vi "Power Off Dut.vi"(8 "error in":errorcluster, 11 "Power Sequencing File Path":path) -> (0 "error out":errorcluster)   [LabVIEW 2023]
uses:
  NI gRPC Device Server - Action.ctl
  <instrlib>/niDCPower/nidcpower.llb/niDCPower gRPC Device Server.ctl
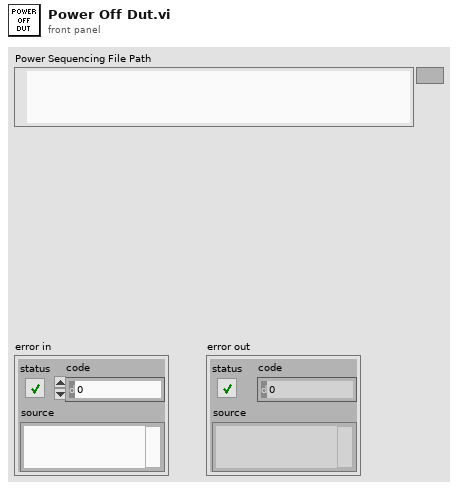
[diagram p1: front panel]
types:
  T1 = typedef "NI gRPC Device Server - Action.ctl" = enum16{"Start Server", "End Server"}
  T2 = typedef "DC Ins Initialize.ctl" = cluster{"Pin Name":string, "Resource Name":refnum<k15>, "Channel":string, "Voltage Range (V)":dbl, "Current Range (A)":dbl}
  T3 = typedef "DC Settings.ctl" = cluster{"Pin Name":string, "Resource Name":refnum<k15>, "Channel":string, "Power-up Seq":u32, "Power-up Voltage (V)":dbl, "Power-down Seq":u32, "Power-down Voltage (V)":dbl, "Current Limit (A)":dbl, "Wait Before Next (ms)":u32}
  T4 = typedef "niDCPower gRPC Device Server.ctl" = cluster{"session name":string, "address (localhost)":string, "port (31763)":u32}
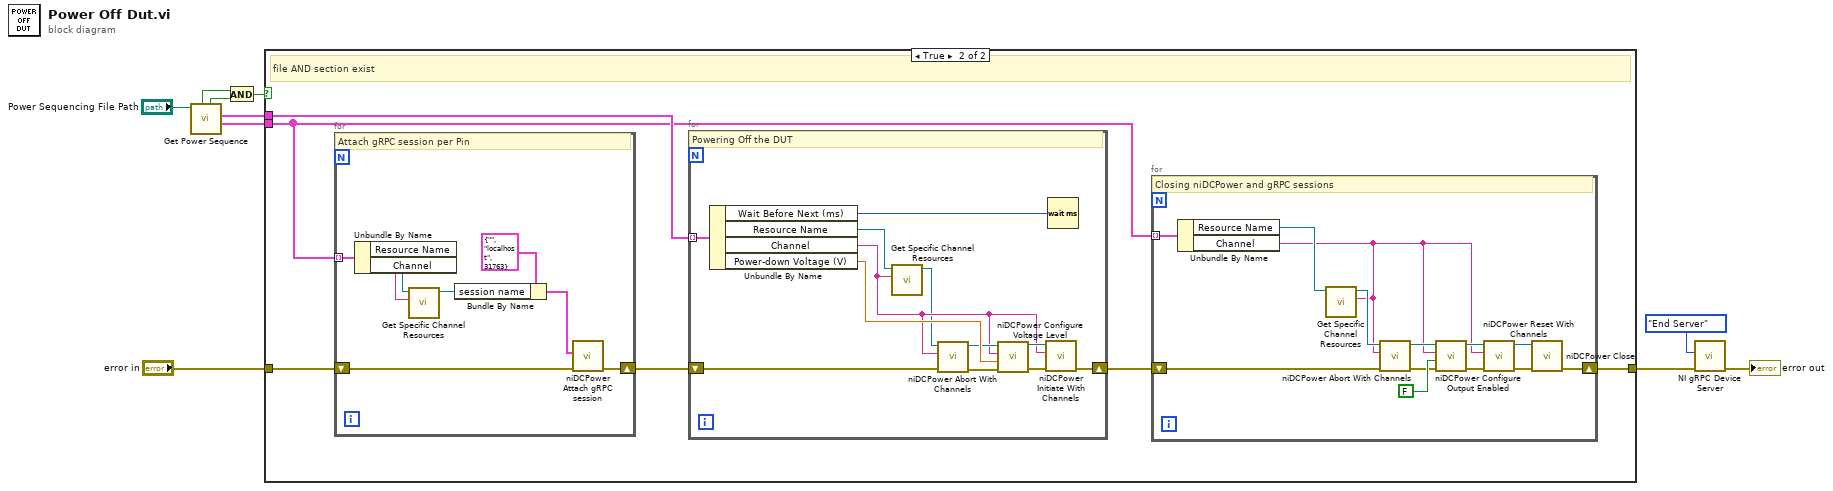
[diagram p0: block diagram]
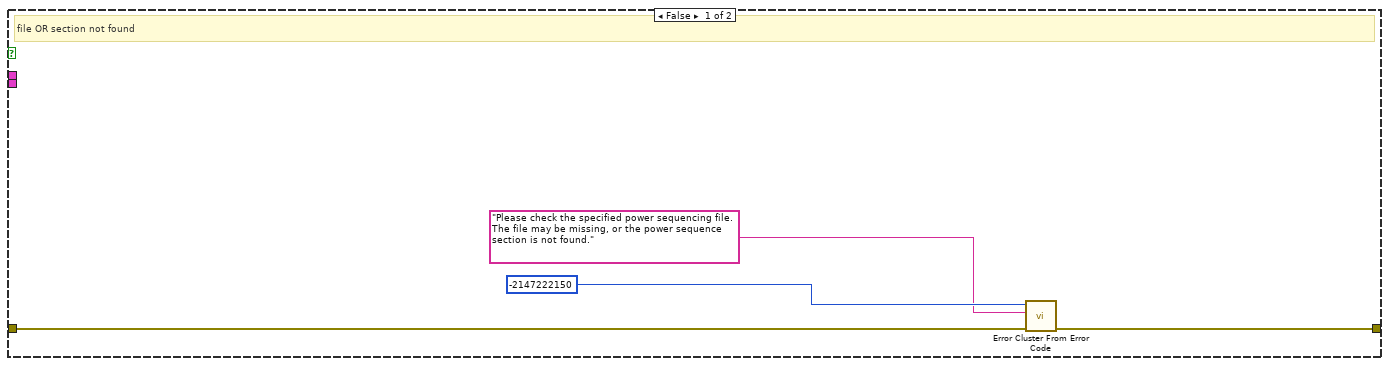
[diagram p2: hidden frame]
diagram:
  n1 = call "Get Power Sequence.vi"("File Path"="Power Sequencing File Path") -> ("SMUs to Initialize (not in order)"=w10:T2[], "Power down Seq"=w9:T3[], "File Exists?"=w6:bool, "Section Exists?"=w5:bool)  [unwired: 6 in, 1 out]
  n2 = And(x=w5, y=w6) -> (x .and. y?=w7:bool)
  n3 = case shown="True" w7 {
    tunnel: w10 -> [_ w16]
    tunnel: w9 -> [_ w20]
    tunnel: "error in" -> [w12 w17]
    tunnel: [w11 w18] -> w3
    frame False {
      # "file OR section not found"
      n4 = call <vilib>:"Error Cluster From Error Code.vi"("error in (no error)"=w12, "error message (\"\")"="Please check the specified power sequencing file. The file may be missing, or the power sequence section is not found.", "error code (0)"=-2147222150) -> ("error out"=w11:errorcluster)  [unwired: 6 in]
    }
    frame True {
      # "file AND section exist"
      n5 = for {
        tunnel: w16 -> [w28] mode=indexing
        shift-right: [w21] -> w15
        shift-left: w17 -> [w22]
        # "Attach gRPC session per Pin"
        n6 = Unbundle By Name(w28) -> ("Resource Name"=w27:refnum<k15>, "Channel"=w26:string)
        n7 = call "Get Specific Channel Resources.vi"("Channel"=w26, "Resource Name"=w27) -> ("Resource Name"=w24:refnum<k15>)  [unwired: 9 in]
        n8 = Bundle By Name(cluster=T4 {"session name"="", "address (localhost)"="localhost", "port (31763)"=31763} ("gRPC options"), "session name"=w24) -> (w23:T4)
        n9 = call <instrlib>:"niDCPower Attach gRPC session.vi"("error in (no error)"=w22, "gRPC options"=w23) -> ("error out"=w21:errorcluster)  [unwired: 8 in, 1 out]
      }
      n10 = for {
        tunnel: w20 -> [w38] mode=indexing
        shift-right: [w33] -> w19
        shift-left: w15 -> [w30]
        # "Powering Off the DUT"
        n11 = Unbundle By Name(w38) -> ("Wait Before Next (ms)"=w39:u32, "Resource Name"=w40:refnum<k15>, "Channel"=w31:string, "Power-down Voltage (V)"=w37:dbl)
        n12 = call "Get Specific Channel Resources.vi"("Channel"=w31, "Resource Name"=w40) -> ("Resource Name"=w29:refnum<k15>)  [unwired: 9 in]
        n13 = call <instrlib>:"niDCPower Abort With Channels.vi"("error in (no error)"=w30, "channel name"=w31, "instrument handle"=w29) -> ("error out"=w36:errorcluster, "instrument handle out"=w35:refnum<k15>)  [unwired: 7 in]
        n14 = call <instrlib>:"niDCPower Configure Voltage Level.vi"("error in (no error)"=w36, "voltage level"=w37, "channel name"=w31, "instrument handle"=w35) -> ("error out"=w34:errorcluster, "instrument handle out"=w32:refnum<k15>)  [unwired: 6 in]
        n15 = call <instrlib>:"niDCPower Initiate With Channels.vi"("error in (no error)"=w34, "channel name"=w31, "instrument handle"=w32) -> ("error out"=w33:errorcluster)  [unwired: 7 in, 1 out]
        n16 = Wait (ms)(milliseconds to wait=w39) -> ()  [unwired: 1 out]
      }
      n17 = for {
        tunnel: w16 -> [w50] mode=indexing
        shift-right: [w41] -> w18
        shift-left: w19 -> [w47]
        # "Closing niDCPower and gRPC sessions"
        n18 = Unbundle By Name(w50) -> ("Resource Name"=w53:refnum<k15>, "Channel"=w42:string)
        n19 = call "Get Specific Channel Resources.vi"("Channel"=w42, "Resource Name"=w53) -> ("Resource Name"=w48:refnum<k15>)  [unwired: 9 in]
        n20 = call <instrlib>:"niDCPower Abort With Channels.vi"("error in (no error)"=w47, "channel name"=w42, "instrument handle"=w48) -> ("error out"=w45:errorcluster, "instrument handle out"=w46:refnum<k15>)  [unwired: 7 in]
        n21 = call <instrlib>:"niDCPower Configure Output Enabled.vi"("error in (no error)"=w45, "output enabled"=FALSE, "channel name"=w42, "instrument handle"=w46) -> ("error out"=w43:errorcluster, "instrument handle out"=w44:refnum<k15>)  [unwired: 6 in]
        n22 = call <instrlib>:"niDCPower Reset With Channels.vi"("error in (no error)"=w43, "channel name"=w42, "instrument handle"=w44) -> ("error out"=w51:errorcluster, "instrument handle out"=w52:refnum<k15>)  [unwired: 7 in]
        n23 = call <instrlib>:"niDCPower Close.vi"("error in (no error)"=w51, "instrument handle"=w52) -> ("error out"=w41:errorcluster)  [unwired: 9 in]
      }
    }
  }
  n24 = call "NI gRPC Device Server.vi"("error in"=w3, "Action"=NI_gRPC_Device_Server_-_Action."End Server") -> ("error out"=→"error out":errorcluster)  [unwired: 9 in]
